vi "LED_KnightRiderCycle.vi"   [LabVIEW 2018]
uses:
  <vilib>/rvi/Emulation/niFpgaGetClockAttributes.vi
  <vilib>/rvi/Emulation/niFpgaSctlEmulationGetInTimedLoop.vi
  <vilib>/rvi/Emulation/niFpgaEmulationReportErrorSimple.vi
  <vilib>/rvi/eio/common/nirviEmuTemplateMethod_errors.vi
  <vilib>/rvi/Emulation/niFpgaCriticalErrorInLSC.vi
  <vilib>/eio/EIONode/EIONode.xnode
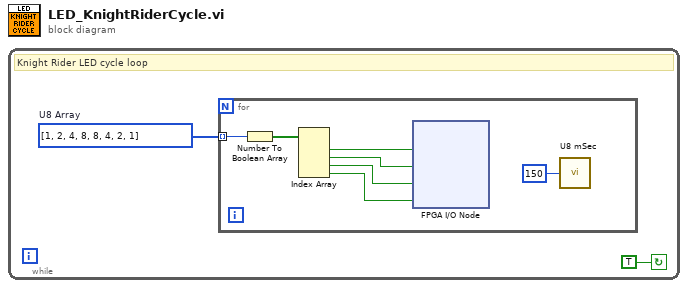
[diagram p0: block diagram]
diagram:
  n1 = while {
    stop <- TRUE continue-if-true
    w1 = u8[] [1, 2, 4, 8, 8, 4, 2, 1]  # U8 Array
    # "Knight Rider LED cycle loop"
    n2 = for {
      tunnel: w1 -> [w9] mode=indexing
      n3 = Number To Boolean Array(number=w9) -> (Boolean array=w8:bool[])
      n4 = Index Array(array=w8) -> (element #1=w7:bool, element #2=w6:bool, element #3=w5:bool, element #4=w4:bool)  [unwired: 4 in]
      n5 = xnode "FPGA I/O Node"("LED0"=w7, "LED1"=w6, "LED2"=w5, "LED3"=w4) -> ()  [unwired: 4 in, 4 out]
      n6 = call "U8 mSec"("Count(mSec)"=u8 150) -> ()  [unwired: 1 out]
    }
  }
